vi "fire actor ui.vi"(11 "Template in":refnum<class "Template.lvclass">) -> ()   [LabVIEW 2020, in "Template.lvlib" / "Template.lvclass"]
uses:
  Template.lvclass
  Template.lvclass/Template.ctl
  accessors/Read This Actor Number.vi
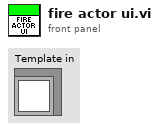
[diagram p1: front panel]
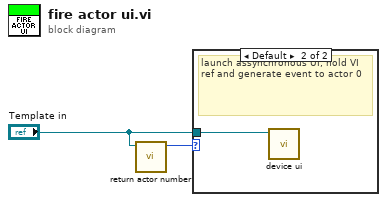
[diagram p0: block diagram]
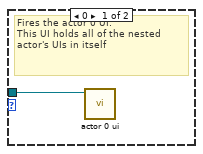
[diagram p2: hidden frame]
diagram:
  n1 = call "return actor number.vi"("Template in"="Template in") -> ("Actor number"=w2:u32)  [unwired: 10 in]
  n2 = case shown="Default" w2 {
    tunnel: "Template in" -> [w3 w4]
    frame 0 {
      # "Fires the actor 0 UI.\nThis UI holds all of the nested actor's UIs in itself"
      n3 = call "actor 0 ui.vi"("Template in"=w3) -> ()  [unwired: 11 in]
    }
    frame Default {
      # "launch assynchronous UI, hold VI ref and generate event to actor 0"
      n4 = call-dynamic "device ui.vi"("Template in"=w4) -> ()  [unwired: 11 in]
    }
  }
